vi "Periodic Tasks.vi"(8 "error in":errorcluster) -> ()   [LabVIEW 2013]
doc: "This VI runs in parallel to other tasks. It can contain as many user-defined periodic loops as you need. These can carry out PID or other sorts of timed response."
uses:
  <vilib>/Rock Robotics/SystemInterfaces/Utilities/FPGA_UtilitiesLED Source.ctl
  <vilib>/Rock Robotics/SystemInterfaces/Utilities/FPGA_UtilitiesLED State.ctl
  Robot Global Data.vi
  <vilib>/Rock Robotics/WPI/Compressor/WPI_CompressorGetSetRefNum.vi
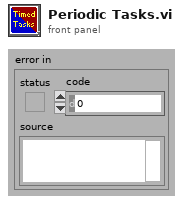
[diagram p1: front panel]
types:
  T1 = typedef "WPI_CompressorDevRef.ctl" = cluster{"DevStatus":errorcluster, "DigitalInputDevRef":T2, "RelayDevRef":T5}
  T2 = typedef "WPI_DigitalInputDevRef.ctl" = cluster{"DevStatus":errorcluster, "DIO Channel":T3, "Digital Module":T4}
  T3 = typedef "FPGA_DIOChannel.ctl" = enum8{"DIO 1", "DIO 2", "DIO 3", "DIO 4", "DIO 5", "DIO 6", "DIO 7", "DIO 8", "DIO 9", "DIO 10", "DIO 11", "DIO 12", "DIO 13", "DIO 14", "Invalid"}
  T4 = typedef "FPGA_TypedefDigitalModule.ctl" = enum16{"Digital Module 1", "Digital Module 2"}
  T5 = typedef "WPI_RelayDevRef.ctl" = cluster{"DevStatus":errorcluster, "Relay Channel":T6, "Digital Module":T4, "Relay Direction":T7}
  T6 = typedef "FPGA_DIORelayChannel.ctl" = enum8{"Relay 1", "Relay 2", "Relay 3", "Relay 4", "Relay 5", "Relay 6", "Relay 7", "Relay 8", "Invalid"}
  T7 = typedef "WPI_RelayDirection.ctl" = enum16{"Both directions", "Forward only", "Reverse only"}
  T8 = typedef "FPGA_UtilitiesLED State.ctl" = enum16{"Off", "On", "Toggle"}
  T9 = typedef "FPGA_UtilitiesLED Source.ctl" = enum16{"User LED", "FPGA LED"}
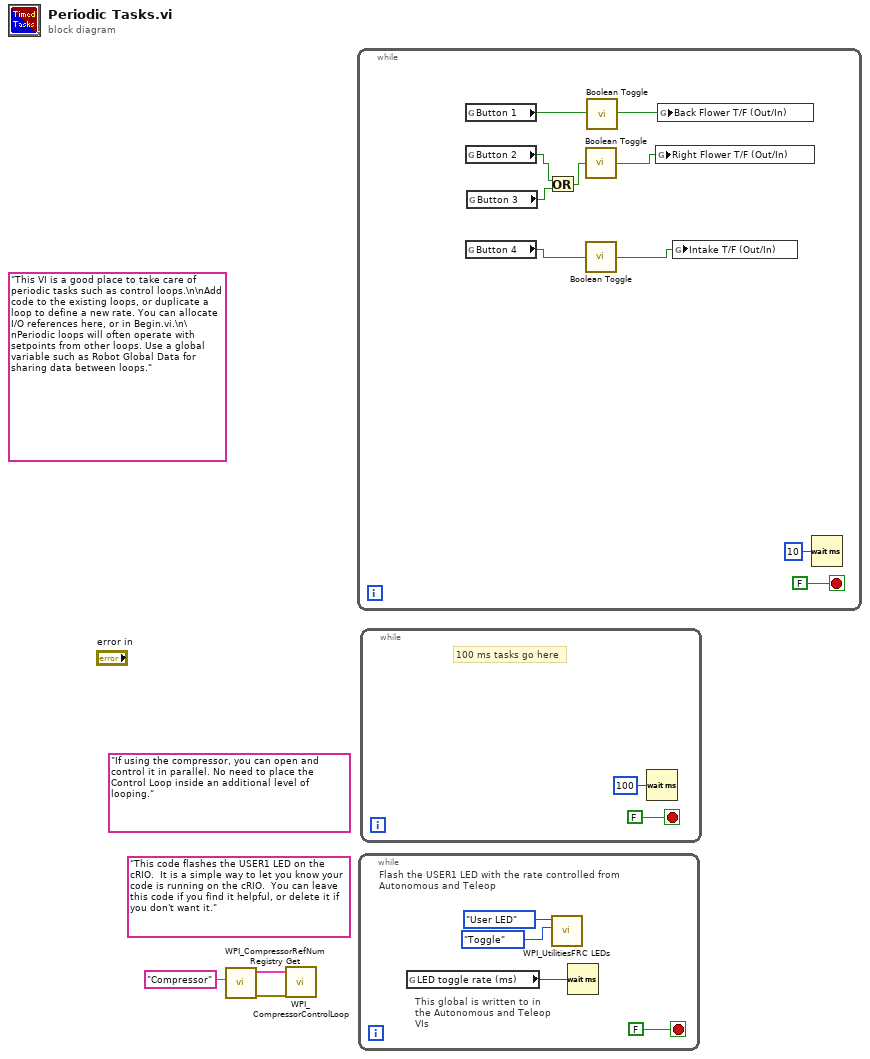
[diagram p0: block diagram]
diagram:
  (unwired) "If using the compressor, you can open and control it in parallel. No need to place the Control Loop inside an additional level of looping."
  (unwired) "This code flashes the USER1 LED on the cRIO.  It is a simple way to let you know your code is running on the cRIO.  You can leave this code if you find it helpful, or delete it if you don't want it."
  (unwired) "This VI is a good place to take care of periodic tasks such as control loops.\n\nAdd code to the existing loops, or duplicate a loop to define a new rate. You can allocate I/O references here, or in Begin.vi.\n\nPeriodic loops will often operate with setpoints from other loops. Use a global variable such as Robot Global Data for sharing data between loops."
  n1 = call <vilib>:"WPI_CompressorRefNum Registry Get.vi"("refnum name"="Compressor") -> ("error out"=w3:errorcluster, "CompressorDevRef"=w2:T1)  [unwired: 9 in]
  n2 = call <vilib>:"WPI_CompressorControlLoop.vi"("error in (no error)"=w3, "CompressorDevRef"=w2) -> ()  [unwired: 10 in]
  n3 = while {
    stop <- FALSE stop-if-true
    n4 = global read "Robot Global Data.vi" "Button 1"() -> (w11:bool)
    n5 = global read "Robot Global Data.vi" "Button 2"() -> (w5:bool)
    n6 = global read "Robot Global Data.vi" "Button 4"() -> (w10:bool)
    n7 = global read "Robot Global Data.vi" "Button 3"() -> (w6:bool)
    n8 = Or(x=w5, y=w6) -> (x .or. y?=w4:bool)
    n9 = call "Boolean Toggle.vi"("Input"=w4) -> ("Output"=w8:bool)
    n10 = call "Boolean Toggle.vi"("Input"=w10) -> ("Output"=w9:bool)
    n11 = call "Boolean Toggle.vi"("Input"=w11) -> ("Output"=w7:bool)
    n12 = global write "Robot Global Data.vi" "Right Flower T/F (Out/In)"(w8) -> ()
    n13 = global write "Robot Global Data.vi" "Back Flower T/F (Out/In)"(w7) -> ()
    n14 = global write "Robot Global Data.vi" "Intake T/F (Out/In)"(w9) -> ()
    n15 = Wait (ms)(milliseconds to wait=u32 10) -> ()  [unwired: 1 out]
  }
  n16 = while {
    stop <- FALSE stop-if-true
    # "This global is written to in the Autonomous and Teleop VIs"
    # "Flash the USER1 LED with the rate controlled from Autonomous and Teleop"
    n17 = global read "Robot Global Data.vi" "LED toggle rate (ms)"() -> (w14:u32)
    n18 = call <vilib>:"WPI_UtilitiesFRC LEDs.vi"("State"=FPGA_UtilitiesLED_State."Toggle", "LED Type"=FPGA_UtilitiesLED_Source."User LED") -> ()  [unwired: 1 in, 9 out]
    n19 = Wait (ms)(milliseconds to wait=w14) -> ()  [unwired: 1 out]
  }
  n20 = while {
    stop <- FALSE stop-if-true
    # "100 ms tasks go here"
    n21 = Wait (ms)(milliseconds to wait=u32 100) -> ()  [unwired: 1 out]
  }
